vi "main.vi"() -> ()   [LabVIEW 2014]
uses:
  <vilib>/Instr/_visa.llb/VISA Configure Serial Port (Instr).vi
  <instrlib>/Hokuyo URG Series/Public/Initialize-Standard.vi
  <vilib>/Utility/file.llb/Write To Spreadsheet File (DBL).vi
  <instrlib>/Hokuyo URG Series/Hokuyo URG Series.lvlib
panel:
  in  "Lidar VISA resource name":refnum<visa-resource-name>="COM3"
  in  "Stop":dbl
  in  "Stop 2":bool
  out "Real iteration angle":dbl
  out "Angle":dbl
  in  "Vertical resolution":dbl
  in  "Motor VISA resource name":refnum<visa-resource-name>
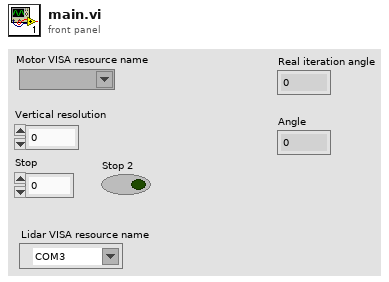
[diagram p1: front panel]
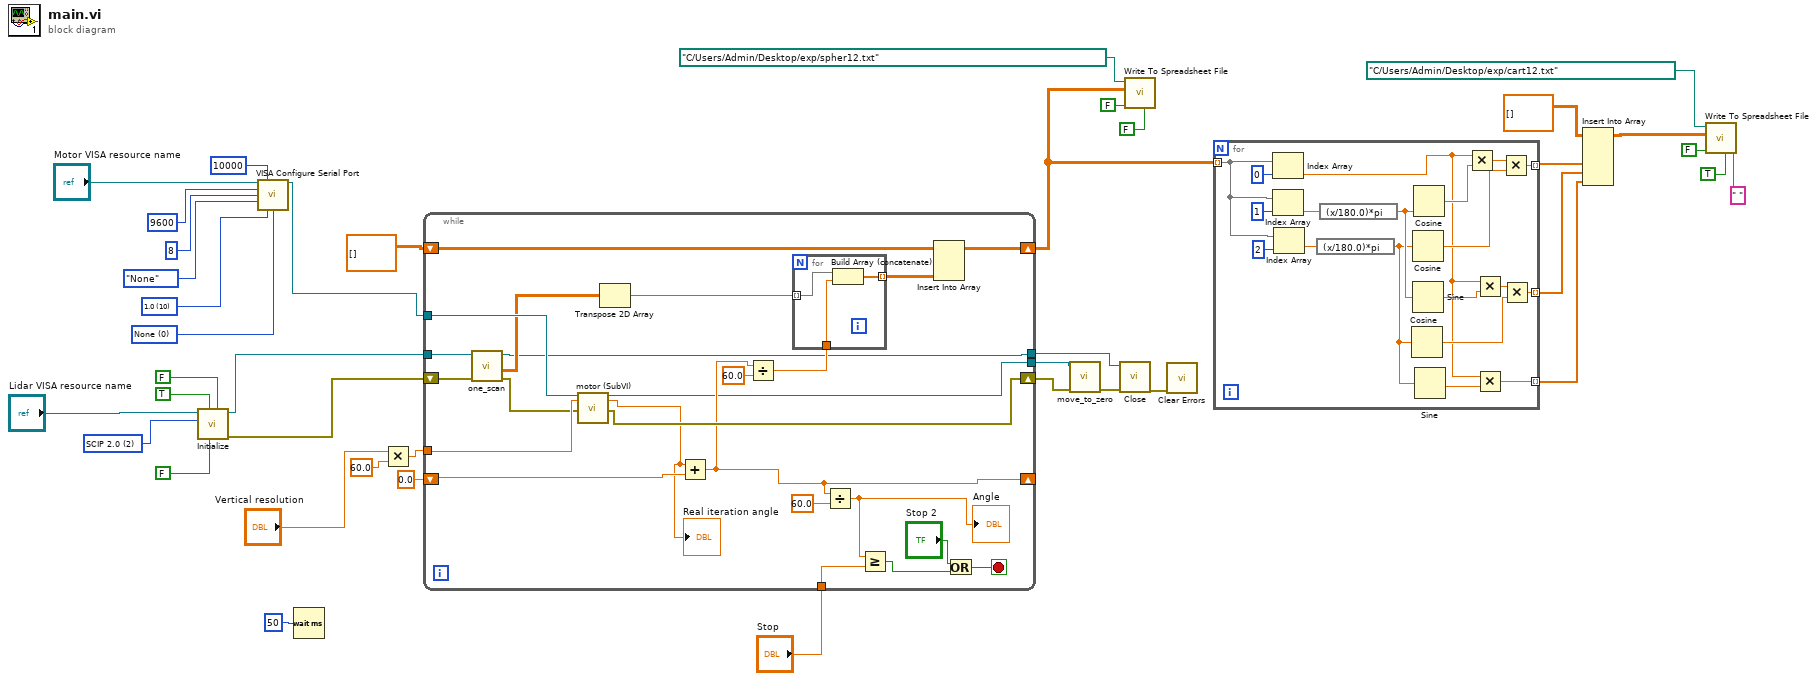
[diagram p0: block diagram]
diagram:
  w14 = u32 2 items=["Convert to Latest", "SCIP 1.1", "SCIP 2.0"] ("Protocol")
  w33 = u16 0 items=["None", "XON/XOFF", "RTS/CTS", "XON/XOFF & RTS/CTS", "DTR/DSR", "XON/XOFF & DTR/DSR"] ("flow control (0:none)")
  w34 = u16 10 items=["1.0"=10, "1.5"=15, "2.0"=20] ("stop bits (10: 1 bit)")
  n1 = call-poly <instrlib>:"Initialize.vi"("Reset? (F: No)"=FALSE ("Reset Instrument (Disabled)"), "Checksum (Disabled)"=FALSE ("Checksum"), "ID Query? (Enabled)"=TRUE ("ID Query?"), "Protocol (2: SCIP 2.0)"=w14, "VISA resource name"="Lidar VISA resource name") -> ("error out"=w12:errorcluster, "VISA resource name out"=w11:refnum<visa-resource-name>)  [unwired: 5 in]
  n2 = call-poly "VISA Configure Serial Port"("VISA resource name"="Motor VISA resource name", "timeout (10sec)"=u32 10000, "baud rate (9600)"=u32 9600, "data bits (8)"=u16 8, "parity (0:none)"=enum16{"None", "Odd", "Even", "Mark", "Space"}."None", "stop bits (10: 1 bit)"=w34, "flow control (0:none)"=w33) -> ("VISA resource name out"=w22:refnum<visa-resource-name>)  [unwired: 7 in, 1 out]
  n3 = Wait (ms)(milliseconds to wait=u32 50) -> ()  [unwired: 1 out]
  n4 = Multiply(x="Vertical resolution", y=60.0) -> (x*y=w31:dbl)
  n5 = while {
    tunnel: w22 -> [w63]
    tunnel: w31 -> [w64]
    shift-right: [w62] -> w23
    shift-left: w12 -> [w43]
    tunnel: "Stop" -> [w56]
    shift-right: [w53] -> _
    shift-left: 0.0 -> [w58]
    shift-right: [w49] -> w18
    shift-left: dbl[][] [] -> [w50]
    tunnel: [w46] -> w24
    tunnel: w11 -> [w42]
    tunnel: [w41] -> w8
    stop <- w59 stop-if-true
    n6 = call "one_scan.vi"("error in (no error)"=w43, "VISA Refnum in"=w42) -> ("error out"=w44:errorcluster, "PhiR Array"=w45:dbl[][], "VISA Refnum out"=w41:refnum<visa-resource-name>)  [unwired: 6 in, 1 out]
    n7 = call "motor (SubVI).vi"("VISA Refnum in"=w63, "step"=w64, "error in (no error)"=w44) -> ("VISA resource name out"=w46:refnum<visa-resource-name>, "Angle"=w47:dbl, "error out"=w62:errorcluster)  [unwired: 14 in]
    "Real iteration angle" <- w47
    n8 = Transpose 2D Array(2D array=w45) -> (transposed array=w51:dbl[][])
    n9 = Add(x=w47, y=w58) -> (x+y=w53:dbl)
    n10 = Divide(x=w53, y=60.0) -> (x/y=w52:dbl)
    n11 = for {
      tunnel: w51 -> [w65] mode=indexing
      tunnel: [w67] -> w48 mode=indexing
      tunnel: w52 -> [w66]
      n12 = Build Array (concatenate)(w65, w66) -> (w67:dbl[])
    }
    n13 = Divide(x=w53, y=60.0) -> (x/y=w55:dbl)
    "Angle" <- w55
    n14 = Greater Or Equal?(x=w55, y=w56) -> (x >= y?=w61:bool)
    n15 = Insert Into Array(array=w50, new element=w48) -> (w49:dbl[][])  [unwired: 2 in]
    n16 = Or(x="Stop 2", y=w61) -> (x .or. y?=w59:bool)
  }
  n17 = call "move_to_zero.vi"("error in (no error)"=w23, "VISA Refnum in"=w24) -> ("error out"=w9:errorcluster)  [unwired: 8 in, 1 out]
  n18 = call <instrlib>:"Close.vi"("error in (no error)"=w9, "VISA resource name"=w8) -> ("error out"=w10:errorcluster)  [unwired: 9 in]
  n19 = call-poly <vilib>:"Write To Spreadsheet File.vi"("transpose? (no:F)"=FALSE, "append to file? (new file:F)"=FALSE, "2D data"=w18, "file path (dialog if empty)"=path "C:/Users/Admin/Desktop/exp/spher12.txt") -> ()  [unwired: 4 in, 1 out]
  n20 = call <vilib>:"Clear Errors.vi"("error in (no error)"=w10) -> ()  [unwired: 5 in, 2 out]
  n21 = for {
    tunnel: w18 -> [w83] mode=indexing
    tunnel: [w79] -> w6 mode=indexing
    tunnel: [w73] -> w4 mode=indexing
    tunnel: [w70] -> w5 mode=indexing
    n22 = Index Array(array=w83, index=0) -> (element=w72:dbl)
    n23 = Index Array(array=w83, index=1) -> (element=w77:dbl)
    n24 = Index Array(array=w83, index=2) -> (element=w78:dbl)
    n25 = expression code="(x/180.0)*pi"(w78) -> (w68:dbl)
    n26 = expression code="(x/180.0)*pi"(w77) -> (w69:dbl)
    n27 = Cosine(x=w68) -> (cos(x)=w74:dbl)
    n28 = Cosine(x=w68) -> (cos(x)=w80:dbl)
    n29 = Sine(x=w69) -> (sin(x)=w76:dbl)
    n30 = Cosine(x=w69) -> (cos(x)=w82:dbl)
    n31 = Sine(x=w68) -> (sin(x)=w71:dbl)
    n32 = Multiply(x=w72, y=w82) -> (x*y=w81:dbl)
    n33 = Multiply(x=w72, y=w76) -> (x*y=w75:dbl)
    n34 = Multiply(x=w72, y=w71) -> (x*y=w70:dbl)
    n35 = Multiply(x=w81, y=w80) -> (x*y=w79:dbl)
    n36 = Multiply(x=w75, y=w74) -> (x*y=w73:dbl)
  }
  n37 = Insert Into Array(array=dbl[][] [], new element #1=w6, new element #2=w4, new element #3=w5) -> (w3:dbl[][])  [unwired: 2 in]
  n38 = call-poly <vilib>:"Write To Spreadsheet File.vi"("delimiter (\\t)"=" " ("delimiter (\\t)"), "transpose? (no:F)"=TRUE, "append to file? (new file:F)"=FALSE, "2D data"=w3, "file path (dialog if empty)"=path "C:/Users/Admin/Desktop/exp/cart12.txt") -> ()  [unwired: 3 in, 1 out]
